vi "MyG#G3Templ_GetAttributesToModify.vi"(0 "reference in":refnum<class "MyG#G3Templ.lvclass">, 3 "timeout in ms (-1)":i32=-1, 5 "error in (no error)":errorcluster) -> (14 "reference out":refnum<class "MyG#G3Templ.lvclass">, 15 "attributes ref":T2, 16 "attributes":T1, 17 "timeout":bool, 19 "error out":errorcluster)   [LabVIEW 2020, in "MyG#G3Templ.lvclass"]
doc: "This VI returns the class attributes associated with the object reference and places a lock on the object. If reference is wired, the class attributes of this class (or sub class) will be returned else the class attributes will default to the class.\n\nIf the object is currently locked for modification by another method, 'Timeout' specifies how long the VI should wait to receive access to the object. The default value waits until the object becomes available.\n\nYou must use this class SetModifiedClassAttributes VI to set the object's data and release the lock."
uses:
  MyG#G3Templ.lvclass
  ObjectAttributesRef.ctl
  protected/ObjectAttributes.ctl
  MyG#G3Templ.lvclass/MyG#G3Templ.ctl
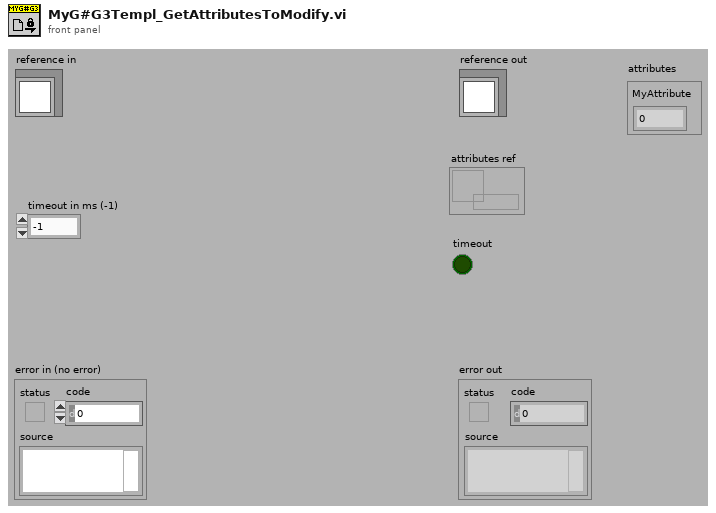
[diagram p1: front panel]
types:
  T1 = typedef "MyG#G3Templ.lvclass/ObjectAttributes.ctl" = cluster{"MyAttribute":dbl}
  T2 = typedef "MyG#G3Templ.lvclass/ObjectAttributesRef.ctl" = refnum<data-value>
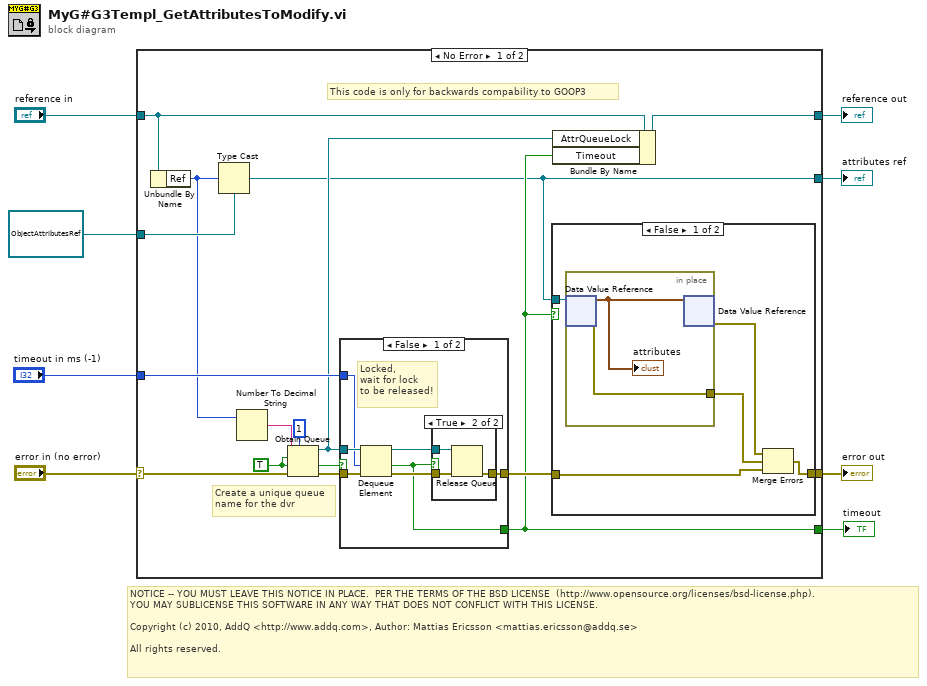
[diagram p0: block diagram]
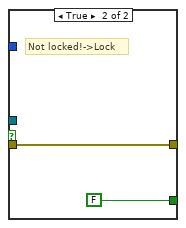
[diagram p3: hidden frame]
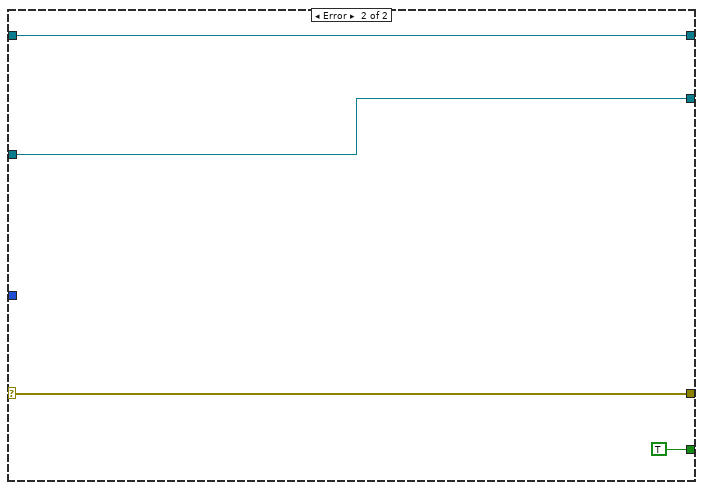
[diagram p5: hidden frame]
diagram:
  # "NOTICE -- YOU MUST LEAVE THIS NOTICE IN PLACE.  PER THE TERMS OF THE BSD LICENSE  (http://www.opensource.org/licenses/bsd-license.php).\nYOU MAY SUBLICENSE THIS SOFTWARE IN ANY WAY THAT DOES NOT CONFLICT WITH THIS LICENSE.\n\nCopyright (c) 2010, AddQ <http://www.addq.com>, Author: Mattias Ericsson <mattias.ericsson@addq.se>\n\nAll rights reserved."
  n1 = case shown="No Error" "error in (no error)" {
    selector: "error in (no error)" -> [w16 w49]
    tunnel: [w24 w49] -> w7
    tunnel: [w14 w48] -> w5
    tunnel: "reference in" -> [w15 w48]
    tunnel: [w9 w46] -> w4
    tunnel: "timeout in ms (-1)" -> [w17 _]
    tunnel: [w12 TRUE ("status")] -> w2
    tunnel: T2 refnum ("attributes ref") -> [w11 w46]
    frame No Error {
      w22 = TRUE ("create if not found? (T)")
      # "Create a unique queue\nname for the dvr"
      # "This code is only for backwards compability to GOOP3"
      n2 = Unbundle By Name(w15) -> ("Ref"=w10:u32)
      n3 = Type Cast(type=w11, x=w10) -> (*(type *) &x=w9:T2)
      n4 = Number To Decimal String(number=w10) -> (decimal integer string=w23:string)  [unwired: 1 in]
      n5 = Obtain Queue(max queue size (-1, unlimited)=1, name (unnamed)=w23, element data type=w22, create if not found? (T)=w22, error in (no error)=w16) -> (queue out=w13:refnum<queue>, created new?=w19:bool, error out=w20:errorcluster)
      n6 = case shown="False" w19 {
        tunnel: w20 -> [w29 w36]
        tunnel: [w28 w36] -> w18
        tunnel: w13 -> [w31 _]
        tunnel: w17 -> [w30 _]
        tunnel: [w25 FALSE ("status")] -> w12
        frame False {
          # "Locked,\nwait for lock\nto be released!"
          n7 = Dequeue Element(queue=w31, timeout in ms (-1)=w30, error in (no error)=w29) -> (queue out=w26:refnum<queue>, timed out?=w25:bool, error out=w27:errorcluster)  [unwired: 1 out]
          n8 = case shown="True" w25 {
            tunnel: [w32 w35] -> w28
            tunnel: w27 -> [w32 w34]
            tunnel: w26 -> [_ w33]
            frame False {
            }
            frame True {
              n9 = Release Queue(queue=w33, error in (no error)=w34) -> (error out=w35:errorcluster)  [unwired: 1 in, 2 out]
            }
          }
        }
        frame True {
          # "Not locked!->Lock"
        }
      }
      n10 = case shown="False" w12 {
        tunnel: w9 -> [w42 _]
        tunnel: w18 -> [w41 w45]
        tunnel: [w38 w45] -> w24
        frame False {
          n11 = in-place {
            in-place-border: [w44] -> w40
            n12 = in-place-dvr #1(w42) -> (w43:T1, w44:errorcluster)
            "attributes" <- w43
            n13 = in-place-dvr #1(w43) -> (w39:errorcluster)  [unwired: 1 out]
          }
          n14 = Merge Errors(w39, w40, w41) -> (w38:errorcluster)
        }
        frame True {
        }
      }
      n15 = Bundle By Name(cluster=w15, "AttrQueueLock"=w13, "Timeout"=w12) -> (w14:refnum<class "MyG#G3Templ.lvclass">)
    }
    frame Error {
    }
  }
  "error out" <- w7
  "reference out" <- w5
  "attributes ref" <- w4
  "timeout" <- w2
